vi "AnalogIntegratorFastOszi_3GHz_NI5771.vi"() -> ()   [LabVIEW 2014]
uses:
  <vilib>/Platform/TimedLoop/XDataNode/timing_clust.ctl
  <vilib>/Platform/TimedLoop/XDataNode/nitl_modes.ctl
  <vilib>/Platform/TimedLoop/XDataNode/wakeup.ctl
  <vilib>/rvi/Emulation/niFpgaGetClockAttributes.vi
  <vilib>/rvi/Emulation/niFpgaSctlEmulationGetInTimedLoop.vi
  <vilib>/rvi/Emulation/niFpgaEmulationReportErrorSimple.vi
  <vilib>/rvi/eio/common/nirviEmuTemplateMethod_errors.vi
  <vilib>/rvi/Emulation/niFpgaCriticalErrorInLSC.vi
  <vilib>/rvi/Emulation/niFpgaEmulationIsFPGAContextNoSignature.vi
  <vilib>/rvi/FIFO/Fifo_Resource/nirvififoEmulationSetSize.vi
  <vilib>/rvi/DataTransferAndStorage/Container/Common/niFpgaContainerGetUniqueNameForEmu.vi
  <vilib>/rvi/FIFO/Fifo_Resource/nirviFifoEmulationQueueMgr.vi
  <instcachedir>/0/nirviFifoEmulationQueueMgr_E5CAEC123FF24DC58D834DCA3CDAA9B5.lvgen/nirviFifoEmulationQueueMgr_E5CAEC123FF24DC58D834DCA3CDAA9B5_004.vi
  <vilib>/rvi/Emulation/niFpgaProcessEmulError.vi
  <vilib>/rvi/errors/niFpgaSetErrorForExecOnDevCompSimple.vi
  <vilib>/rvi/eio/common/nirviEmuReportErrorAndStop.vi
  <vilib>/rvi/FIFO/Fifo_Resource/nirvififoEmulationDetermineInputValidOut.vi
  <vilib>/rvi/FIFO/Fifo_Resource/nirvififoEmulationCreateLock.vi
  <vilib>/rvi/FIFO/Fifo_Resource/nirvififoEmulationObtainLock.vi
  <vilib>/rvi/FIFO/Fifo_Resource/nirvififoEmulationReleaseLock.vi
  <vilib>/rvi/occurrence/nirviWaitOnOccurrenceBase.vi
  <vilib>/rvi/errors/nirviReportUnexpectedCaseInternalError.vi
  <vilib>/rvi/errors/nirviReportUnexpectedCaseInternalError (U32).vi
  <vilib>/rvi/interface/RandomDataEmulation/niFpgaRandomDataHandleErrors.vi
  <vilib>/eio/EIONode/EIONode.xnode
  <vilib>/rvi/DataTransferAndStorage/Container/XNode/niFpgaContainer.xnode
  <vilib>/rvi/FIFO/Fifo_Resource/nirvififoEmulationClear.vi
  <vilib>/Platform/TimedLoop/XDataNode/XDataNode.xnode
  <vilib>/rvi/FIFO/Fifo_Resource/nirvififoEmulationWrite.vi
  <vilib>/rvi/FIFO/Fifo_Resource/nirvififoEmulationRead.vi
  <vilib>/rvi/interface/RandomDataEmulation/nirviRandomDataFpgaReadWriteTemplate.vi
  <vilib>/Platform/TimedLoop/XDataNode/XDNodeRunTimeDep.lvlib
panel:
  in  "Baseline U8":u8
  in  "Acquire continuously":bool
  in  "Clear Interloop FIFO":bool
  out "InterloopFIFO Timeout":bool
  out "ToHostCh1FIFO Overflow":bool
  in  "Acquire":bool
  out "InterloopFIFO Overflow":bool
  out "Acquiring":bool
  out "IO Module\\AI Over Range":bool
  in  "Samples to acquire":u32=10000 caption="Samples per pixel Acq"
  in  "User Command Commit":bool
  in  "User Command":u8
  out "User Command Idle":bool
  out "User Command Status":u8
  in  "User Data 0":u16
  in  "User Data 1":u8
  out "PLL Locked":bool
  out "User Error":bool
  out "Configured?":bool
  # "5771 IO module configuration"
  # "Analog integrator Fast Oszi mode"
  # "Acquisition control"
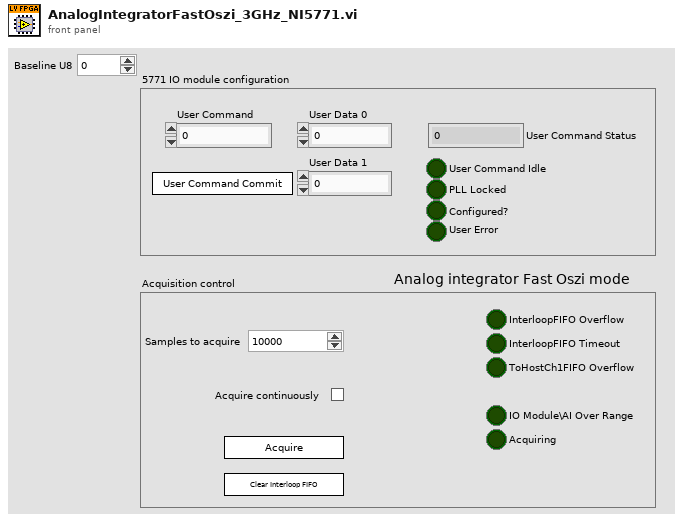
[diagram p1: front panel]
types:
  T1 = typedef "XDNodeRunTimeDep.lvlib/timing_clust.ctl" = cluster{"Expected End [f-1]":u64, "Actual End [f-1]":u64, "Finished Late? [f-1]":bool, "Expected End [i-1]":u64, "Actual End [i-1]":u64, "Finished Late? [i-1]":bool, "Expected Start [i]":u64, "Actual Start [i]":u64, "Expected Start [f]":u64, "Actual Start [f]":u64, "Source Name":string, "Structure Name":string, "Period":i64, "Deadline":i64, "Offset":i64, "Start":i64, "Priority":i32, "Timeout":i32, "Mode":T2, "Wakeup Reason":T3, "Error":errorcluster, "Source Type":string, "Secondary Source Type":string, "Global End Time":u64, "Global Start Time":u64, "Frame Duration":u64, "Iteration Duration":u64, "Assigned CPU":i32, "I/O Scan Engine Mode":u32}
  T2 = typedef "XDNodeRunTimeDep.lvlib/nitl_modes.ctl" = enum32{"No Change", "Process missed periods, maintain original phase", "Discard missed periods, maintain original phase", "Process missed periods, ignore original phase", "Discard missed periods, ignore original phase"}
  T3 = typedef "XDNodeRunTimeDep.lvlib/wakeup.ctl" = enum32{"Normal", "Aborted", "Asynchronous wakeup", "Timing source error", "Timed loop error", "Timeout"}
  T4 = cluster{"Data U64 1":u64, "IO Module\\Synchronous Trigger Input":u8, "Data U64 2":u64}
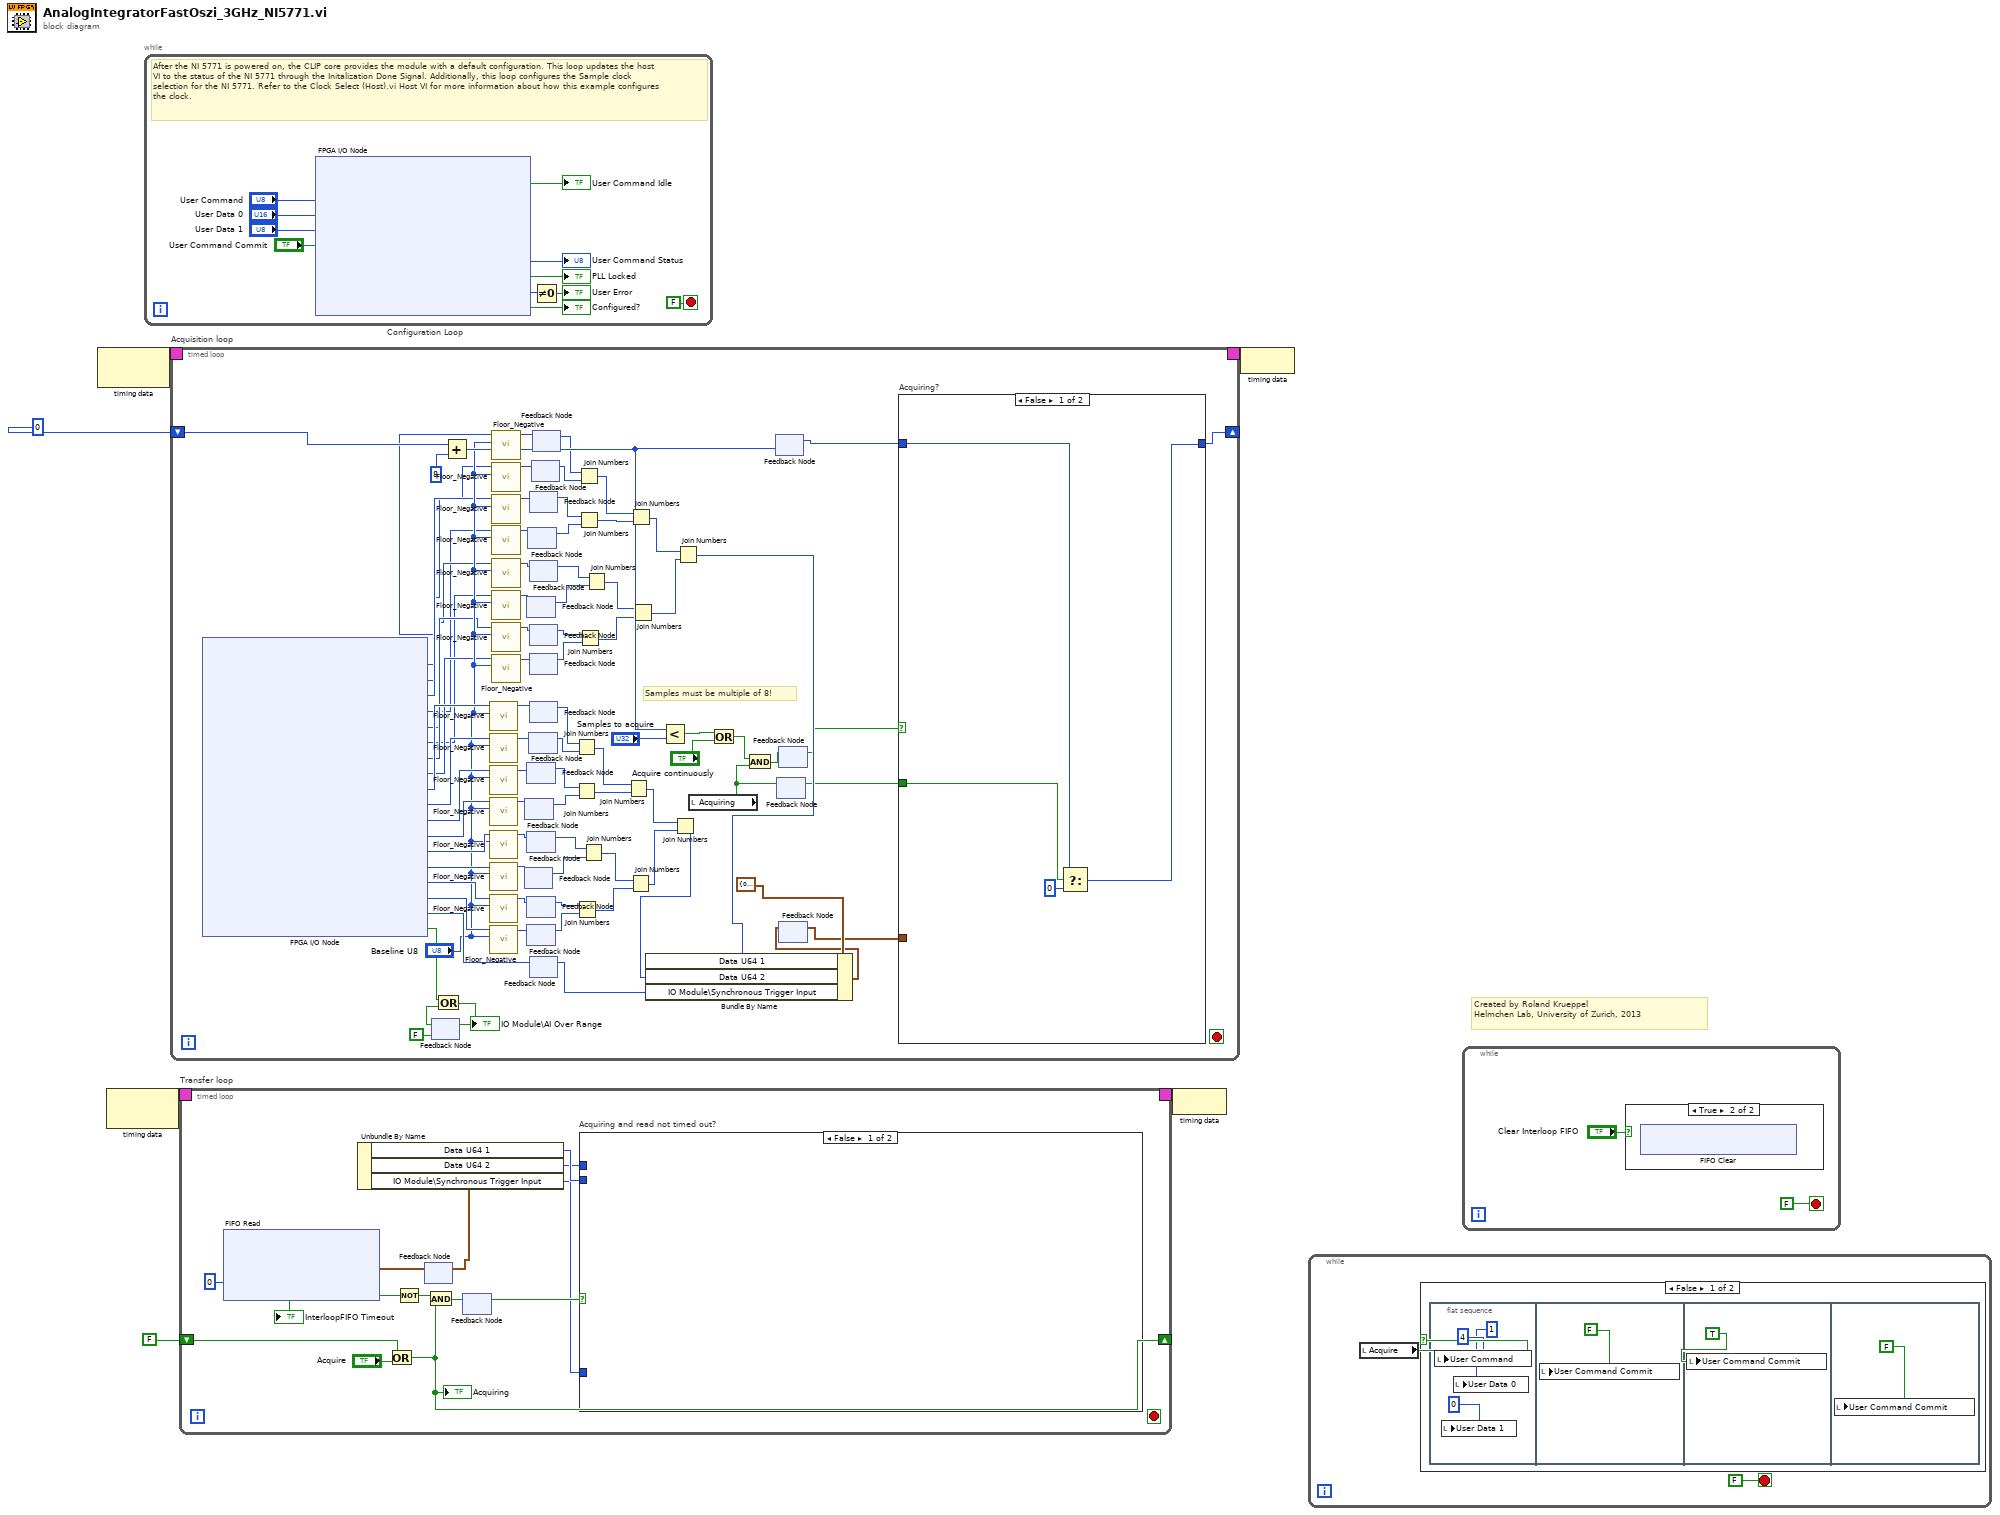
[diagram p0: block diagram]
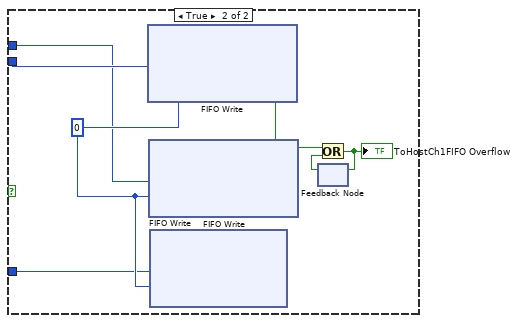
[diagram p4: hidden frame]
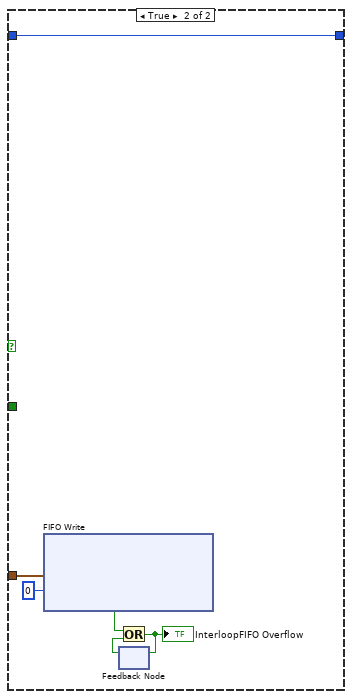
[diagram p5: hidden frame]
diagram:
  # "Created by Roland Krueppel\nHelmchen Lab, University of Zurich, 2013"
  n1 = node-c288() -> (w6:T1)  [unwired: 1 in]
  n2 = node-c288() -> (w3:T1)  [unwired: 1 in]
  n3 = while "Configuration Loop" {
    stop <- FALSE stop-if-true
    # "After the NI 5771 is powered on, the CLIP core provides the module with a default configuration. This loop updates the host VI to the status of the NI 5771 through the Initalization Done Signal. Additionally, this loop configures the Sample clock selection for the NI 5771. Refer to the Clock Select (Host).vi Host VI for more information about how this example configures the clock."
    n4 = xnode "FPGA I/O Node"("IO Module\\User Command"="User Command", "IO Module\\User Data 0"="User Data 0", "IO Module\\User Data 1"="User Data 1", "IO Module\\User Command Commit"="User Command Commit") -> ("IO Module\\User Command Idle"=→"User Command Idle":bool, "IO Module\\User Command Status"=→"User Command Status":u8, "IO Module\\PLL Locked"=→"PLL Locked":bool, "IO Module\\User Error"=w12:u8, "IO Module\\Initialization Done"=→"Configured?":bool)  [unwired: 9 in, 9 out]
    n5 = Not Equal To 0?(x=w12) -> (x != 0?=→"User Error":bool)
  }
  n6 = timed-loop "Acquisition loop" {
    timing: w6 -> [_]
    timing-out: [_] -> w5
    shift-right: [w20] -> _
    shift-left: u32 0 ("t") -> [w96]
    stop <- _ stop-if-true
    # "Samples must be multiple of 8!"
    n7 = xnode "FPGA I/O Node"() -> ("IO Module\\AI 1 Data N-7"=w28:u8, "IO Module\\AI 0 Data N-7"=w29:u8, "IO Module\\AI 1 Data N-6"=w30:u8, "IO Module\\AI 0 Data N-6"=w31:u8, "IO Module\\AI 1 Data N-5"=w32:u8, "IO Module\\AI 0 Data N-5"=w33:u8, "IO Module\\AI 1 Data N-4"=w34:u8, "IO Module\\AI 0 Data N-4"=w35:u8, "IO Module\\AI 1 Data N-3"=w83:u8, "IO Module\\AI 0 Data N-3"=w82:u8, "IO Module\\AI 1 Data N-2"=w81:u8, "IO Module\\AI 0 Data N-2"=w80:u8, "IO Module\\AI 1 Data N-1"=w79:u8, "IO Module\\AI 0 Data N-1"=w76:u8, "IO Module\\AI 1 Data N"=w77:u8, "IO Module\\AI 0 Data N"=w78:u8, "IO Module\\Synchronous Trigger Input"=w75:u8, "IO Module\\AI Over Range"=w102:bool)  [unwired: 18 in, 18 out]
    n8 = feedback #1(FALSE) -> (w101:bool)
    n9 = Or(x=w102, y=w101) -> (x .or. y?=w100:bool)
    "IO Module\\AI Over Range" <- w100
    n10 = feedback-in #1(w100) -> ()
    n11 = Add(x=w96, y=u32 8) -> (x+y=w89:u32)
    n12 = call "Floor_Negative.vi"("Baseline U8"="Baseline U8", "Input Value"=w83) -> ("Output Value"=w74:u8)  [unwired: 9 in]
    n13 = call "Floor_Negative.vi"("Baseline U8"="Baseline U8", "Input Value"=w82) -> ("Output Value"=w72:u8)  [unwired: 9 in]
    n14 = call "Floor_Negative.vi"("Baseline U8"="Baseline U8", "Input Value"=w81) -> ("Output Value"=w71:u8)  [unwired: 9 in]
    n15 = call "Floor_Negative.vi"("Baseline U8"="Baseline U8", "Input Value"=w80) -> ("Output Value"=w70:u8)  [unwired: 9 in]
    n16 = call "Floor_Negative.vi"("Baseline U8"="Baseline U8", "Input Value"=w79) -> ("Output Value"=w69:u8)  [unwired: 9 in]
    n17 = call "Floor_Negative.vi"("Baseline U8"="Baseline U8", "Input Value"=w76) -> ("Output Value"=w68:u8)  [unwired: 9 in]
    n18 = call "Floor_Negative.vi"("Baseline U8"="Baseline U8", "Input Value"=w77) -> ("Output Value"=w67:u8)  [unwired: 9 in]
    n19 = call "Floor_Negative.vi"("Baseline U8"="Baseline U8", "Input Value"=w78) -> ("Output Value"=w66:u8)  [unwired: 9 in]
    n20 = call "Floor_Negative.vi"("Baseline U8"="Baseline U8", "Input Value"=w28) -> ("Output Value"=w43:u8)  [unwired: 9 in]
    n21 = call "Floor_Negative.vi"("Baseline U8"="Baseline U8", "Input Value"=w29) -> ("Output Value"=w45:u8)  [unwired: 9 in]
    n22 = call "Floor_Negative.vi"("Baseline U8"="Baseline U8", "Input Value"=w30) -> ("Output Value"=w46:u8)  [unwired: 9 in]
    n23 = call "Floor_Negative.vi"("Baseline U8"="Baseline U8", "Input Value"=w31) -> ("Output Value"=w47:u8)  [unwired: 9 in]
    n24 = call "Floor_Negative.vi"("Baseline U8"="Baseline U8", "Input Value"=w32) -> ("Output Value"=w48:u8)  [unwired: 9 in]
    n25 = call "Floor_Negative.vi"("Baseline U8"="Baseline U8", "Input Value"=w33) -> ("Output Value"=w49:u8)  [unwired: 9 in]
    n26 = call "Floor_Negative.vi"("Baseline U8"="Baseline U8", "Input Value"=w34) -> ("Output Value"=w50:u8)  [unwired: 9 in]
    n27 = call "Floor_Negative.vi"("Baseline U8"="Baseline U8", "Input Value"=w35) -> ("Output Value"=w51:u8)  [unwired: 9 in]
    n28 = feedback #2() -> (w63:u8)  [unwired: 1 in]
    n29 = feedback-in #2(w68) -> ()
    n30 = feedback #3() -> (w61:u8)  [unwired: 1 in]
    n31 = feedback-in #3(w70) -> ()
    n32 = feedback #4() -> (w54:u8)  [unwired: 1 in]
    n33 = feedback-in #4(w49) -> ()
    n34 = feedback #5() -> (w60:u8)  [unwired: 1 in]
    n35 = feedback-in #5(w71) -> ()
    n36 = feedback #6() -> (w62:u8)  [unwired: 1 in]
    n37 = feedback-in #6(w69) -> ()
    n38 = feedback #7() -> (w64:u8)  [unwired: 1 in]
    n39 = feedback-in #7(w67) -> ()
    n40 = feedback #8() -> (w65:u8)  [unwired: 1 in]
    n41 = feedback-in #8(w66) -> ()
    n42 = feedback #9() -> (w56:u8)  [unwired: 1 in]
    n43 = feedback-in #9(w47) -> ()
    n44 = feedback #10() -> (w59:u8)  [unwired: 1 in]
    n45 = feedback-in #10(w72) -> ()
    n46 = feedback #11() -> (w57:u8)  [unwired: 1 in]
    n47 = feedback-in #11(w46) -> ()
    n48 = feedback #12() -> (w55:u8)  [unwired: 1 in]
    n49 = feedback-in #12(w48) -> ()
    n50 = feedback #13() -> (w53:u8)  [unwired: 1 in]
    n51 = feedback-in #13(w50) -> ()
    n52 = feedback #14() -> (w52:u8)  [unwired: 1 in]
    n53 = feedback-in #14(w51) -> ()
    n54 = feedback #15() -> (w73:u8)  [unwired: 1 in]
    n55 = feedback-in #15(w74) -> ()
    n56 = feedback #16() -> (w27:u8)  [unwired: 1 in]
    n57 = feedback-in #16(w75) -> ()
    n58 = feedback #17() -> (w58:u8)  [unwired: 1 in]
    n59 = feedback-in #17(w45) -> ()
    n60 = feedback #18() -> (w44:u8)  [unwired: 1 in]
    n61 = feedback-in #18(w43) -> ()
    n62 = Join Numbers(hi=w73, lo=w59) -> ((hi.lo)=w95:u16)
    n63 = Join Numbers(hi=w60, lo=w61) -> ((hi.lo)=w94:u16)
    n64 = Join Numbers(hi=w64, lo=w65) -> ((hi.lo)=w92:u16)
    n65 = Join Numbers(hi=w44, lo=w58) -> ((hi.lo)=w37:u16)
    n66 = Join Numbers(hi=w57, lo=w56) -> ((hi.lo)=w38:u16)
    n67 = Join Numbers(hi=w53, lo=w52) -> ((hi.lo)=w40:u16)
    n68 = Join Numbers(hi=w62, lo=w63) -> ((hi.lo)=w93:u16)
    n69 = Join Numbers(hi=w55, lo=w54) -> ((hi.lo)=w39:u16)
    n70 = Join Numbers(hi=w95, lo=w94) -> ((hi.lo)=w91:u32)
    n71 = Join Numbers(hi=w93, lo=w92) -> ((hi.lo)=w90:u32)
    n72 = Join Numbers(hi=w37, lo=w38) -> ((hi.lo)=w41:u32)
    n73 = Join Numbers(hi=w39, lo=w40) -> ((hi.lo)=w42:u32)
    n74 = Less?(x=w89, y="Samples to acquire") -> (x < y?=w86:bool)
    n75 = Join Numbers(hi=w91, lo=w90) -> ((hi.lo)=w22:u64)
    n76 = Join Numbers(hi=w41, lo=w42) -> ((hi.lo)=w23:u64)
    n77 = Bundle By Name(cluster=T4 {"Data U64 1"=0, "IO Module\\Synchronous Trigger Input"=0, "Data U64 2"=0} ("Element"), "Data U64 1"=w23, "Data U64 2"=w22, "IO Module\\Synchronous Trigger Input"=w27) -> (w25:T4)
    n78 = local read "Acquiring"() -> (w87:bool)
    n79 = Or(x=w86, y="Acquire continuously") -> (x .or. y?=w84:bool)
    n80 = And(x=w84, y=w87) -> (x .and. y?=w88:bool)
    n81 = feedback #19() -> (w21:u32)  [unwired: 1 in]
    n82 = feedback-in #19(w89) -> ()
    n83 = feedback #20() -> (w18:bool)  [unwired: 1 in]
    n84 = feedback-in #20(w87) -> ()
    n85 = feedback #21() -> (w19:bool)  [unwired: 1 in]
    n86 = feedback-in #21(w88) -> ()
    n87 = feedback #22() -> (w24:T4)  [unwired: 1 in]
    n88 = feedback-in #22(w25) -> ()
    n89 = case "Acquiring?" shown="False" w19 {
      tunnel: [w105 w107] -> w20
      tunnel: w24 -> [_ w108]
      tunnel: w21 -> [w103 w107]
      tunnel: w18 -> [w104 _]
      frame False {
        n90 = Select(t=w103, s=w104, f=u32 0 ("t")) -> (s? t:f=w105:u32)
      }
      frame True {
        n91 = xnode ("FIFO Write")("Element"=w108, "Timeout"=0) -> ("Timed Out?"=w111:bool)  [unwired: 1 in, 1 out]
        n92 = feedback #23() -> (w109:bool)  [unwired: 1 in]
        n93 = Or(x=w111, y=w109) -> (x .or. y?=w110:bool)
        "InterloopFIFO Overflow" <- w110
        n94 = feedback-in #23(w110) -> ()
      }
    }
  }
  n95 = timed-loop "Transfer loop" {
    timing: w3 -> [_]
    timing-out: [_] -> w2
    shift-right: [w124] -> _
    shift-left: FALSE -> [w122]
    stop <- _ stop-if-true
    n96 = xnode ("FIFO Read")("Timeout"=0) -> ("Element"=w121:T4, "Timed Out?"=w126:bool)  [unwired: 1 in, 1 out]
    "InterloopFIFO Timeout" <- w126
    n97 = Or(x=w122, y="Acquire") -> (x .or. y?=w124:bool)
    "Acquiring" <- w124
    n98 = Not(x=w126) -> (.not. x?=w125:bool)
    n99 = feedback-in #24(w121) -> ()
    n100 = feedback #24() -> (w118:T4)  [unwired: 1 in]
    n101 = Unbundle By Name(w118) -> ("Data U64 1"=w117:u64, "Data U64 2"=w116:u64, "IO Module\\Synchronous Trigger Input"=w115:u8)
    n102 = And(x=w125, y=w124) -> (x .and. y?=w120:bool)
    n103 = feedback #25() -> (w119:bool)  [unwired: 1 in]
    n104 = feedback-in #25(w120) -> ()
    n105 = case "Acquiring and read not timed out?" shown="False" w119 {
      tunnel: w117 -> [_ w130]
      tunnel: w116 -> [_ w129]
      tunnel: w115 -> [_ w128]
      frame False {
      }
      frame True {
        w131 = 0 ("Timeout")
        n106 = xnode ("FIFO Write")("Element"=w130, "Timeout"=w131) -> ("Timed Out?"=w133:bool)  [unwired: 1 in, 1 out]
        n107 = xnode ("FIFO Write")("Element"=w129, "Timeout"=w131) -> ()  [unwired: 1 in, 2 out]
        n108 = xnode ("FIFO Write")("Element"=w128, "Timeout"=w131) -> ()  [unwired: 1 in, 2 out]
        n109 = feedback #26() -> (w132:bool)  [unwired: 1 in]
        n110 = Or(x=w133, y=w132) -> (x .or. y?=w134:bool)
        "ToHostCh1FIFO Overflow" <- w134
        n111 = feedback-in #26(w134) -> ()
      }
    }
  }
  n112 = node-c288(w2) -> ()
  n113 = node-c288(w5) -> ()
  n114 = while {
    stop <- FALSE stop-if-true
    n115 = local read "Acquire"() -> (w137:bool)
    n116 = case shown="False" w137 {
      frame False {
        n117 = flat-sequence {
          frame #0 {
            n118 = local write "User Command"(i16 4) -> ()
            n119 = local write "User Data 1"(i16 0) -> ()
            n120 = local write "User Data 0"(i16 1) -> ()
          }
          frame #1 {
            n121 = local write "User Command Commit"(FALSE) -> ()
          }
          frame #2 {
            n122 = local write "User Command Commit"(TRUE) -> ()
          }
          frame #3 {
            n123 = local write "User Command Commit"(FALSE) -> ()
          }
        }
      }
      frame True {
      }
    }
  }
  n124 = while {
    stop <- FALSE stop-if-true
    n125 = case shown="True" "Clear Interloop FIFO" {
      frame False {
      }
      frame True {
        n126 = xnode ("FIFO Clear")() -> ()  [unwired: 1 in, 1 out]
      }
    }
  }
